vi "Current_Filepath.vi"(0 "Filename in":path, 1 "Data Type":string="Calibrations") -> (2 "Filename Out":path)   [LabVIEW 2010]
uses:
  Globals/Meas_global.vi
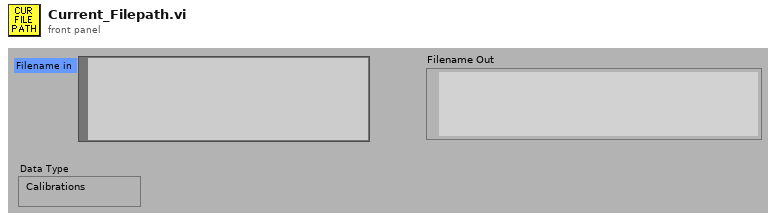
[diagram p1: front panel]
types:
  T1 = typedef "Post_Process.ctl" = enum16{"Take New Data", "Post Process Raw Data File"}
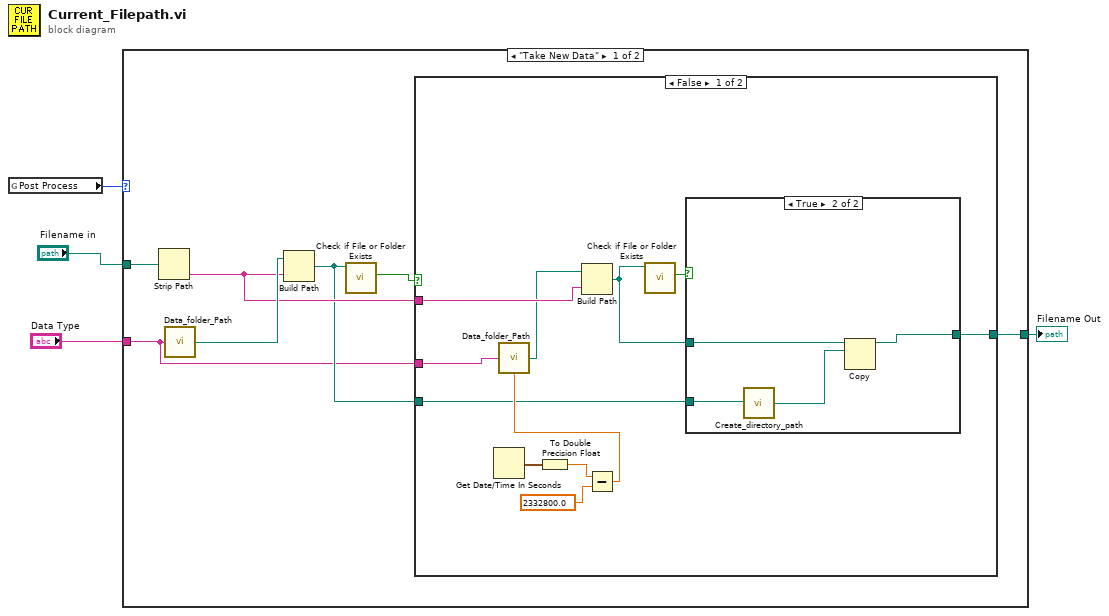
[diagram p0: block diagram]
diagram:
  n1 = global read "Meas_global.vi" "Post Process"() -> (w1:T1)
  n2 = case shown="\"Take New Data\"" w1 {
    tunnel: "Filename in" -> [w11 w29]
    tunnel: "Data Type" -> [w5 _]
    tunnel: [w6 w29] -> w2
    frame "Take New Data" {
      n3 = Strip Path(path=w11) -> (name=w8:string)  [unwired: 1 out]
      n4 = call "Data_folder_Path.vi"("Data Type"=w5) -> ("Data Folder"=w10:path)  [unwired: 1 in]
      n5 = Build Path(base path=w10, name or relative path=w8) -> (appended path=w7:path)
      n6 = call <vilib>:"Check if File or Folder Exists.vi"("path"=w7) -> ("file or folder exists?"=w9:bool)  [unwired: 1 in, 9 out]
      n7 = case shown="False" w9 {
        tunnel: w5 -> [w22 _]
        tunnel: w8 -> [w17 _]
        tunnel: w7 -> [w14 w28]
        tunnel: [w12 w28] -> w6
        frame False {
          n8 = Get Date/Time In Seconds() -> (seconds since 1Jan1904=w21:timestamp)
          n9 = To Double Precision Float(number=w21) -> (double precision float=w20:dbl)
          n10 = Subtract(x=w20, y=2332800.0) -> (x-y=w18:dbl)
          n11 = call "Data_folder_Path.vi"("seconds"=w18, "Data Type"=w22) -> ("Data Folder"=w15:path)
          n12 = Build Path(base path=w15, name or relative path=w17) -> (appended path=w13:path)
          n13 = call <vilib>:"Check if File or Folder Exists.vi"("path"=w13) -> ("file or folder exists?"=w16:bool)  [unwired: 1 in, 9 out]
          n14 = case shown="True" w16 {
            tunnel: w13 -> [_ w27]
            tunnel: w14 -> [w23 w25]
            tunnel: [w23 w26] -> w12
            frame False {
            }
            frame True {
              n15 = call "Create_directory_path.vi"("Path name"=w25) -> ("Path name Out"=w24:path)
              n16 = Copy(10:w24, 11:w27) -> (3:w26:path)  [unwired: 3 in, 2 out]
            }
          }
        }
        frame True {
        }
      }
    }
    frame "Post Process Raw Data File" {
    }
  }
  "Filename Out" <- w2
